vi "rhoplusdot_growth.vi"(5 "rho- sat in":dbl[](array[numeric]), 7 "rho+ sat in":dbl[](array[numeric]), 8 "Sat pol in":dbl, 9 "rho- in":dbl[](array[numeric]), 10 "rho0 in":dbl[](array[numeric]), 11 "rho+ in":dbl[](array[numeric])) -> (3 "rho+ dot out":dbl[](array[numeric]))   [LabVIEW 2018]
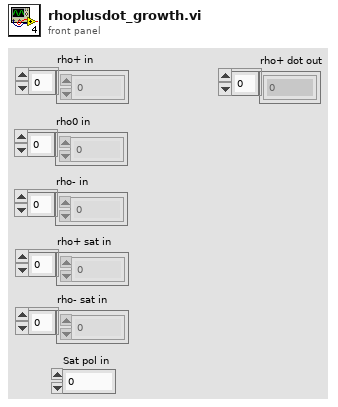
[diagram p1: front panel]
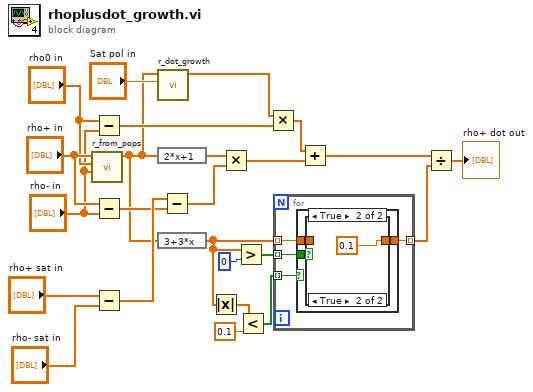
[diagram p0: block diagram]
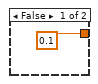
[diagram p3: hidden frame]
diagram:
  n1 = call "r_from_pops.vi"("rho- in"="rho- in", "rho0 in"="rho0 in", "rho+ in"="rho+ in") -> ("r array out"=w5:dbl[])  [unwired: 8 in]
  n2 = Subtract(x="rho0 in", y="rho- in") -> (x-y=w11:dbl[])
  n3 = Subtract(x="rho+ in", y="rho- in") -> (x-y=w19:dbl[])
  n4 = Subtract(x="rho+ sat in", y="rho- sat in") -> (x-y=w20:dbl[])
  n5 = call "r_dot_growth.vi"("Sat pol in"="Sat pol in", "r array in"=w5) -> ("r dot out"=w14:dbl[])  [unwired: 9 in]
  n6 = expression code="2*x+1"(w5) -> (w17:dbl[])
  n7 = expression code="3+3*x"(w5) -> (w4:dbl[])
  n8 = Subtract(x=w20, y=w19) -> (x-y=w18:dbl[])
  n9 = Absolute Value(x=w4) -> (abs(x)=w3:dbl[])
  n10 = Multiply(x=w17, y=w18) -> (x*y=w16:dbl[])
  n11 = Greater?(x=w4, y=0) -> (0:w8:bool[])
  n12 = Less?(x=w3, y=0.1) -> (x < y?=w1:bool[])
  n13 = Multiply(x=w14, y=w11) -> (x*y=w10:dbl[])
  n14 = for {
    tunnel: w8 -> [w28] mode=indexing
    tunnel: w4 -> [w27] mode=indexing
    tunnel: [w26] -> w7 mode=indexing
    tunnel: w1 -> [w25] mode=indexing
    n15 = case shown="True" w25 {
      tunnel: w28 -> [_ w32]
      tunnel: w27 -> [w29 w31]
      tunnel: [w29 w30] -> w26
      frame False {
      }
      frame True {
        n16 = case shown="True" w32 {
          tunnel: w31 -> [_ _]
          tunnel: [0.1 0.1] -> w30
          frame False {
          }
          frame True {
          }
        }
      }
    }
  }
  n17 = Add(x=w10, y=w16) -> (x+y=w15:dbl[])
  n18 = Divide(x=w15, y=w7) -> (x/y=→"rho+ dot out":dbl[])
